vi "Value Tree to Variant.vi"(8 "error in (no error)":errorcluster, 11 "XML in":string) -> (0 "error out":errorcluster, 3 "Value Tree":T1)   [LabVIEW 2018, in "XML Config.lvlib"]
doc: "\"XML in\" is a description of a LabVIEW control (typically a cluster of controls).\nThis VI produces an array row for each primitive control (i.e. not a cluster) with the name path for the control and the value of the control.\n\nFor instance if a cluster named \"Cluster A\" has a numeric named \"numeric B\" and a sub cluster named \"sub cluster\" and a string in the sub cluster named \"string 1\",\nthen the 2D string array output would be something like:\n\nCluster A, numeric B\nCluster A, sub cluster, string 1"
uses:
  XML Config.lvlib
panel:
  out "Name Path":string[][](array[string])
  out "x >= 0?":bool
  out "Values":string[](array[string])
  out "Name Paths":cluster{"Name Path":string[]}[](array[cluster])
  out "Array 2":string[](array[string])
  out "Array":string[](array[string])
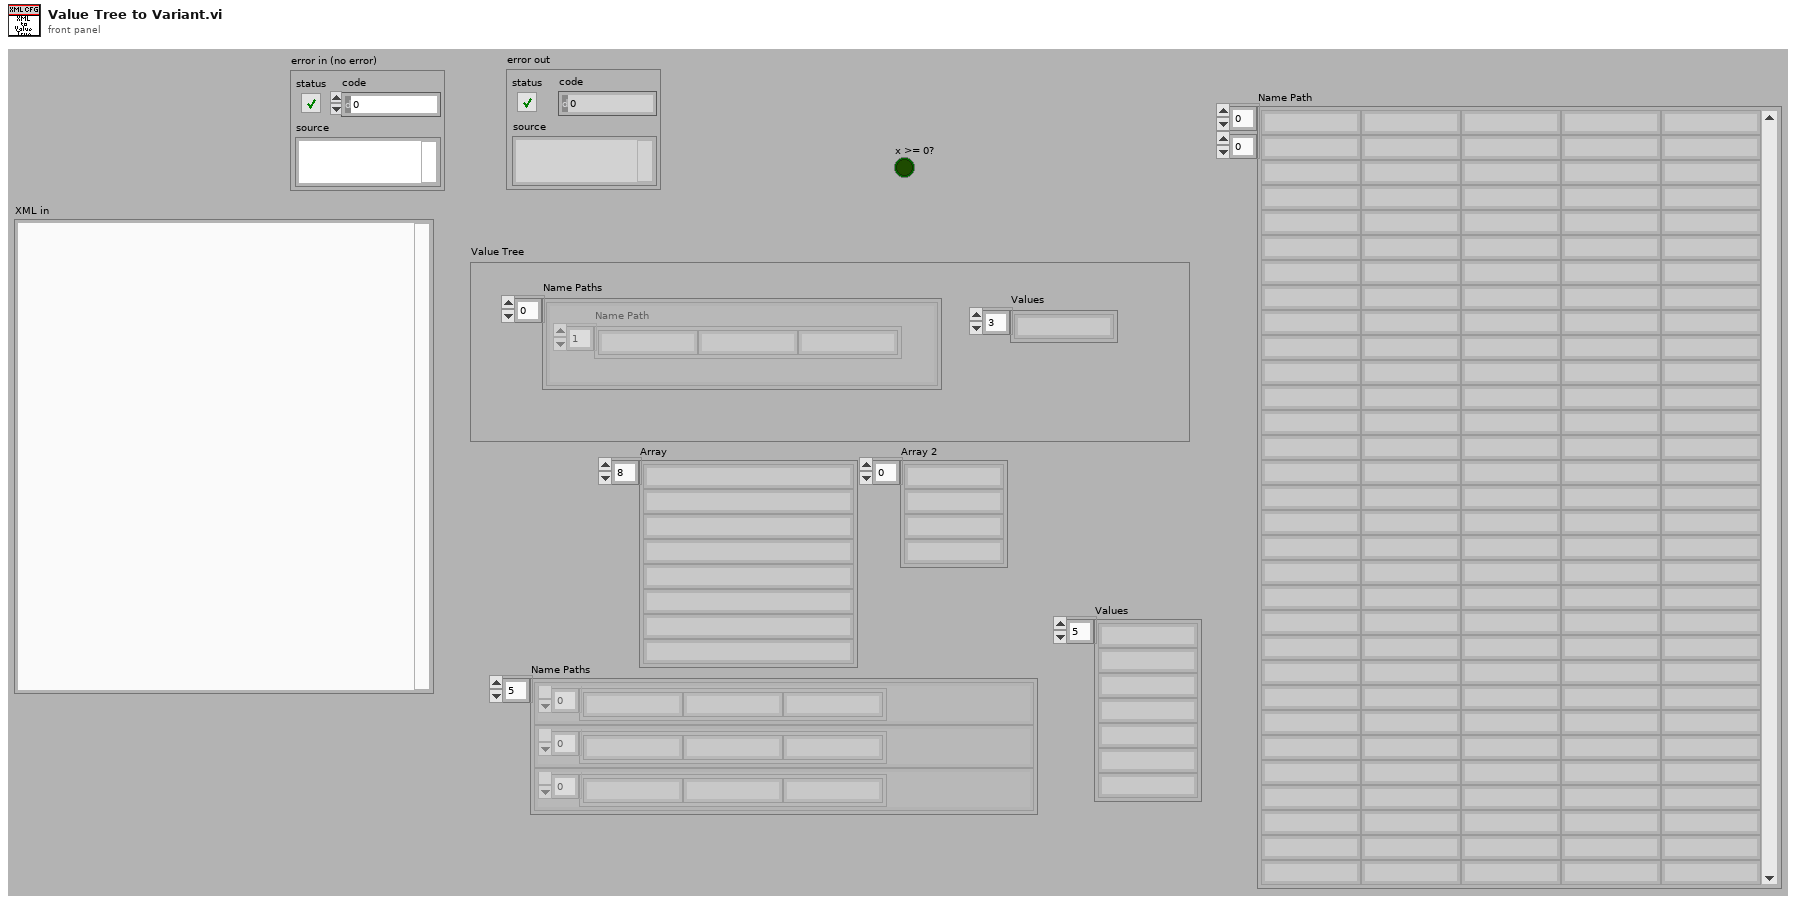
[diagram p1: front panel]
types:
  T1 = cluster{"Name Paths":cluster{"Name Path":string[]}[], "Values":string[]}
  T2 = cluster{cluster{"Name Path":string[]}[], string[]}
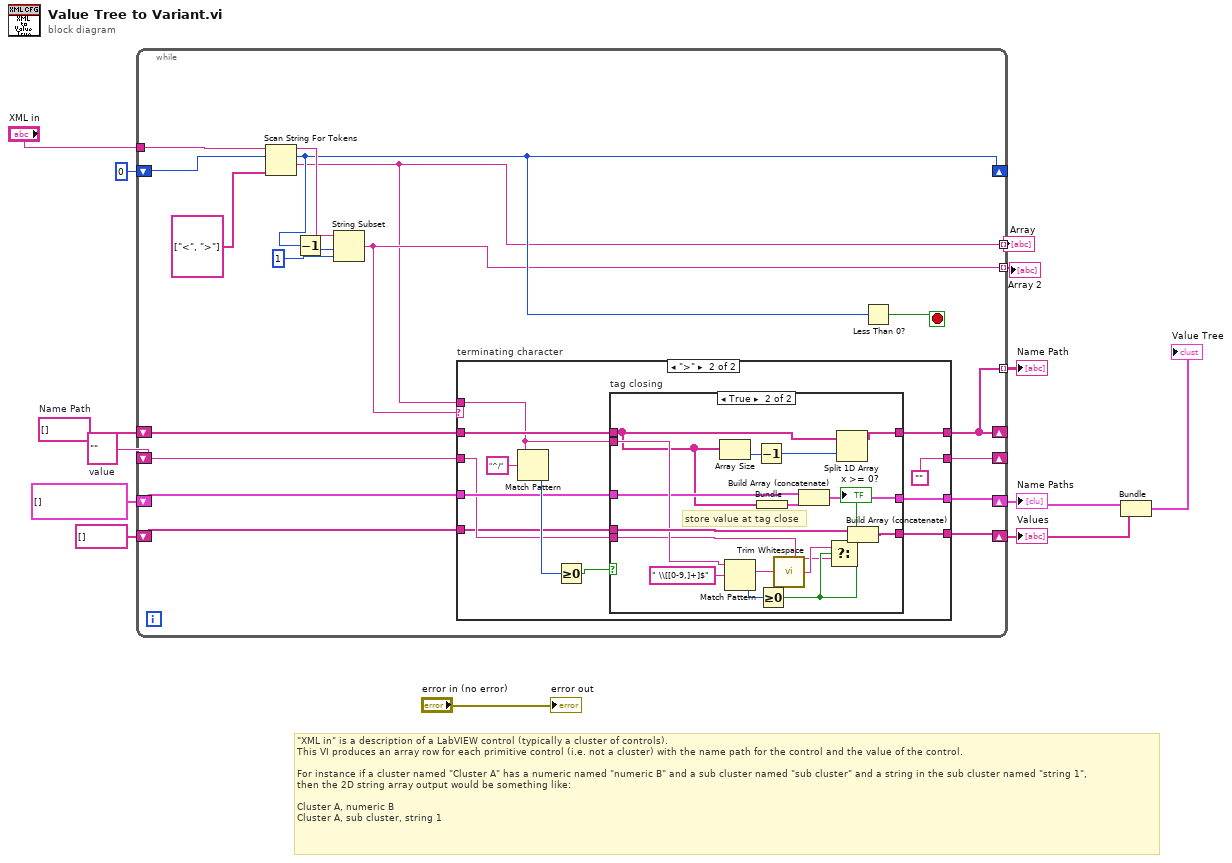
[diagram p0: block diagram]
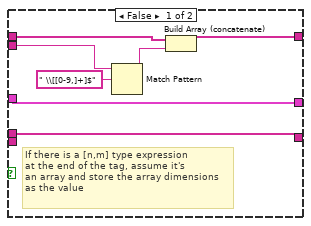
[diagram p3: hidden frame]
diagram:
  w8 = ""  # value
  w9 = string[] []  # Name Path
  # "\"XML in\" is a description of a LabVIEW control (typically a cluster of controls).\nThis VI produces an array row for each primitive control (i.e. not a cluster) with the name path for the control and the value of the control.\n\nFor instance if a cluster named \"Cluster A\" has a numeric named \"numeric B\" and a sub cluster named \"sub cluster\" and a string in the sub cluster named \"string 1\",\nthen the 2D string array output would be something like:\n\nCluster A, numeric B\nCluster A, sub cluster, string 1"
  n1 = while {
    tunnel: "XML in" -> [w31]
    shift-right: [w25] -> _
    shift-left: 0 ("offset past token") -> [w30]
    tunnel: [w15] -> w11 mode=indexing
    tunnel: [w16] -> w10 mode=indexing
    shift-right: [w14] -> _
    shift-left: w9 -> [w23]
    shift-right: [w22] -> _
    shift-left: w8 -> [w21]
    shift-right: [w20] -> w5
    shift-left: cluster{"Name Path":string[]}[] [] -> [w19]
    shift-right: [w18] -> w4
    shift-left: string[] [] -> [w17]
    tunnel: [w14] -> w2 mode=indexing
    stop <- w29 stop-if-true
    n2 = Scan String For Tokens(6:string[] ["<", ">"] ("delimiters (\\s,\\t,\\r,\\n)"), 8:w30, 9:w31) -> (1:w15:string, 2:w25:i32, 3:w27:string)  [unwired: 3 in, 1 out]
    n3 = Decrement(x=w25) -> (x-1=w24:i32)
    n4 = String Subset(string=w27, offset (0)=w24, length (rest)=1 ("length (rest)")) -> (substring=w16:string)
    n5 = case "terminating character" shown="\">\"" w16 {
      tunnel: w23 -> [w35 w44]
      tunnel: w15 -> [w32 w42]
      tunnel: [w35 w43] -> w14
      tunnel: [w32 ""] -> w22
      tunnel: w21 -> [_ w38]
      tunnel: [w34 w41] -> w20
      tunnel: w19 -> [w34 w40]
      tunnel: [w33 w39] -> w18
      tunnel: w17 -> [w33 w37]
      frame "False", Default {
      }
      frame ">" {
        n6 = Match Pattern(string=w42, regular expression="^/") -> (offset past match=w46:i32)  [unwired: 1 in, 3 out]
        n7 = Greater Or Equal To 0?(x=w46) -> (x >= 0?=w45:bool)
        n8 = case "tag closing" shown="True" w45 {
          tunnel: w44 -> [w54 w55]
          tunnel: [w49 w69] -> w43
          tunnel: w42 -> [w51 w64]
          tunnel: [w48 w56] -> w41
          tunnel: w40 -> [w48 w57]
          tunnel: [w53 w68] -> w39
          tunnel: w38 -> [_ w60]
          tunnel: w37 -> [w53 w67]
          frame False {
            # "If there is a [n,m] type expression\nat the end of the tag, assume it's\nan array and store the array dimensions\nas the value"
            n9 = Match Pattern(string=w51, regular expression=" \\[[0-9,]+]$") -> (before substring=w50:string)  [unwired: 1 in, 3 out]
            n10 = Build Array (concatenate)(w54, w50) -> (w49:string[])
          }
          frame True {
            # "store value at tag close"
            n11 = Array Size(array=w55) -> (size(s)=w71:i32)
            n12 = Match Pattern(string=w64, regular expression=" \\[[0-9,]+]$") -> (match substring=w65:string, offset past match=w63:i32)  [unwired: 1 in, 2 out]
            n13 = Decrement(x=w71) -> (x-1=w70:i32)
            n14 = Bundle("Name Path"=w55) -> (w58:cluster{"Name Path":string[]})  [unwired: 1 in]
            n15 = Greater Or Equal To 0?(x=w63) -> (x >= 0?=w62:bool)
            "x >= 0?" <- w62
            n16 = call <vilib>:"Trim Whitespace.vi"("string"=w65) -> ("trimmed string"=w61:string)  [unwired: 1 in]
            n17 = Build Array (concatenate)(w57, w58) -> (w56:cluster{"Name Path":string[]}[])
            n18 = Select(t=w61, s=w62, f=w60) -> (s? t:f=w59:string)
            n19 = Split 1D Array(array=w55, index=w70) -> (first subarray=w69:string[])  [unwired: 1 out]
            n20 = Build Array (concatenate)(w67, w59) -> (w68:string[])
          }
        }
      }
    }
    n21 = Less Than 0?(x=w25) -> (x < 0?=w29:bool)
  }
  "Array" <- w11
  "Array 2" <- w10
  "Name Paths" <- w5
  "Values" <- w4
  "Name Path" <- w2
  n22 = Bundle(w5, w4) -> (→"Value Tree":T2)  [unwired: 1 in]
  "error out" <- "error in (no error)"
